vi "Configure Instrument.vi"(8 "error in (no error)":errorcluster, 11 "Instrument in":refnum<class "Instrument.lvclass">) -> (0 "error out":errorcluster, 3 "Instrument out":refnum<class "Instrument.lvclass">)   [LabVIEW 2016, in "Instrument.lvclass"]
uses:
  Instrument.lvclass
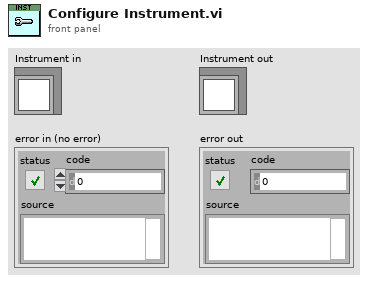
[diagram p1: front panel]
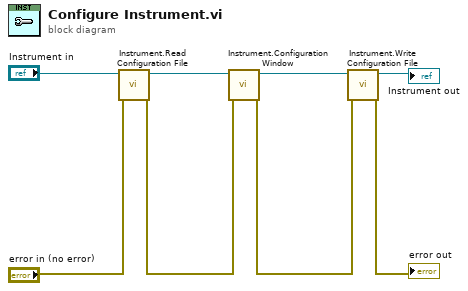
[diagram p0: block diagram]
diagram:
  n1 = call-dynamic "Instrument.Read Configuration File.vi"("error in (no error)"="error in (no error)", "Instrument in"="Instrument in") -> ("error out"=w2:errorcluster, "Instrument out"=w1:refnum<class "Instrument.lvclass">)  [unwired: 8 in]
  n2 = call-dynamic "Instrument.Configuration Window.vi"("error in (no error)"=w2, "Instrument"=w1) -> ("error out"=w4:errorcluster, "Instrument out"=w3:refnum<class "Instrument.lvclass">)  [unwired: 8 in]
  n3 = call-dynamic "Instrument.Write Configuration File.vi"("error in (no error)"=w4, "Instrument in"=w3) -> ("error out"=→"error out":errorcluster, "Instrument out"=→"Instrument out":refnum<class "Instrument.lvclass">)  [unwired: 8 in]
